vi "THzTimeScan_830_PSD_TA_170120.vi"(0 "input":T1={"Step Number"=0, "Step"=0.0, "Start Position"=0.0, "Time-out"=0, "Lockin Address"="", "Short term \nAverage#"=0, 0, "ESP300 Axis"=0, "Value"="", "Delay"=0.0, "Delay2"=0.0, "savepath"=path "", "Power meter"={"ConexPSD Reference"=refnum, "error out"={"status"=FALSE, "code"=0, "source"=""}, "Component ID"=1}}) -> (1 "loop stop":bool, 2 "x-axis":sgl[](array[numeric]), 3 "y-axis":dbl[](array[numeric]), 4 "ext. out":cluster{dbl[], dbl[], dbl[], dbl[], string[]})   [LabVIEW 2010]
uses:
  <vilib>/Utility/file.llb/Write To Spreadsheet File (string).vi
  C:/Users/NBTP/Desktop/Tai Anh/5. Tools Project/LabVIEW/노트북LabVIEW/THz Time/THz Time(SR830_VC_CONEXAGP_nPt_Shot202_2Pt__LGS/Dll/Newport.CONEXPSD.CommandInterface.DLL
  5. Tools Project/LabVIEW/노트북LabVIEW/THz Time/THz Time(SR830_VC_CONEXAGP_nPt_Shot202_2Pt__LGS/Dll/Newport.CONEXPSD.CommandInterface.DLL
panel:
  out "Y position":dbl(graph)
  out "X position":dbl(graph)
  out "Power":dbl(graph)
  out "Y pos.":dbl
  out "X pos.":dbl
  out "Pow.":dbl
  out "Array":dbl[](array[numeric])
  out "String":string
  out "Read position":bool
  out "Ask position":bool
  out "Move delay":bool
  out "Read830":bool
  out "Command":string
  out "THz Signal Graph":dbl(graph)
  in  "loop stop":bool
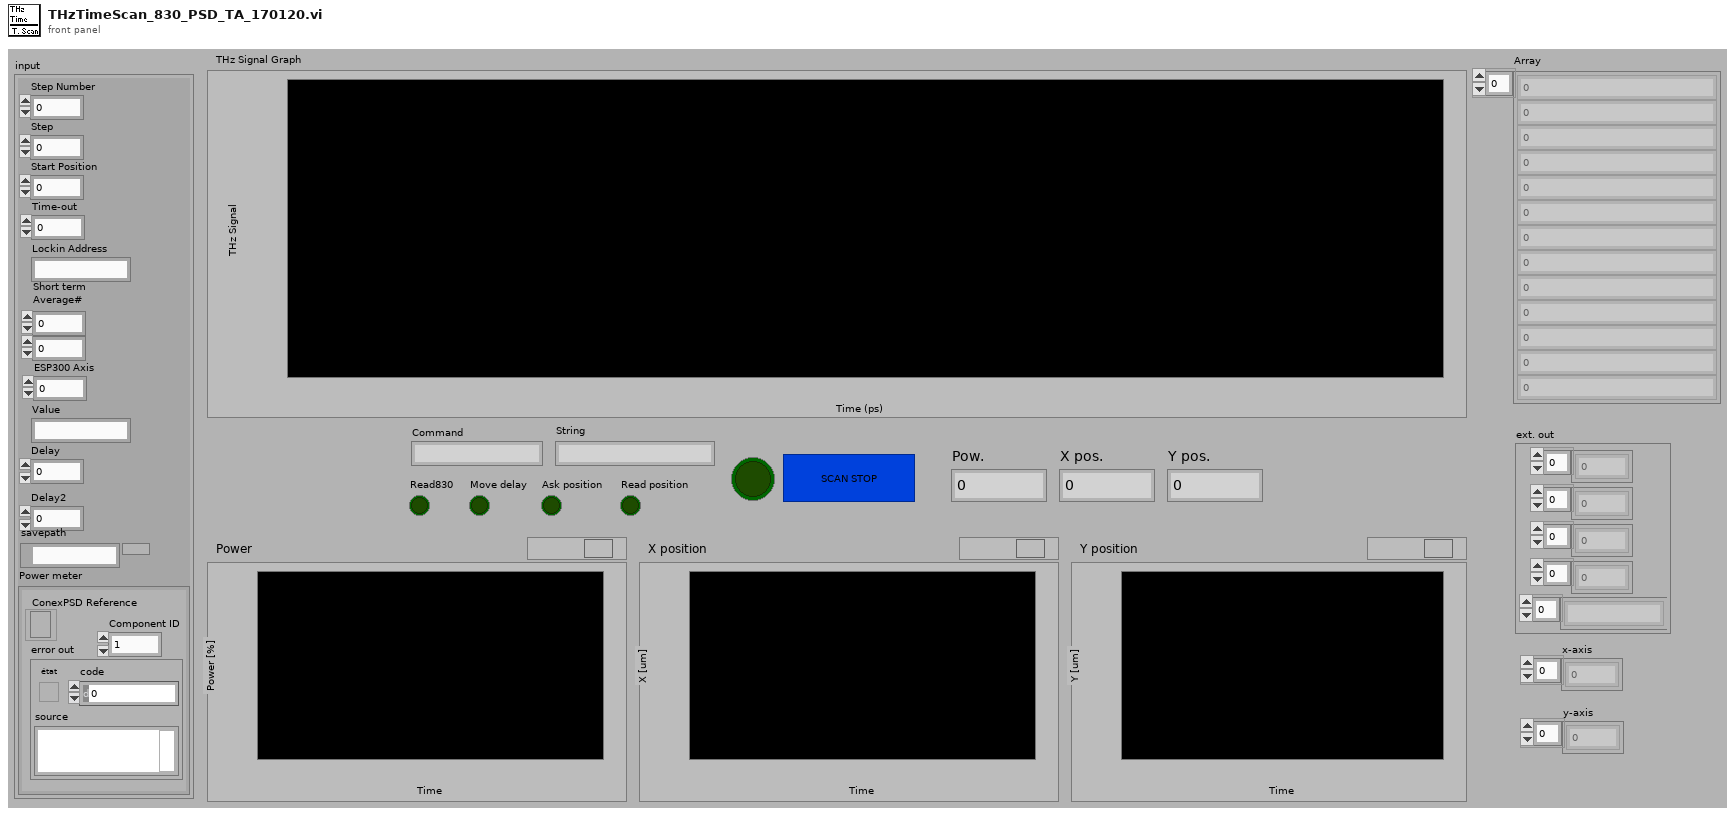
[diagram p1: front panel]
types:
  T1 = cluster{"Step Number":i32, "Step":sgl, "Start Position":sgl, "Time-out":i32, "Lockin Address":string, "Short term \nAverage#":i8, i32, "ESP300 Axis":i8, "Value":string, "Delay":dbl, "Delay2":dbl, "savepath":path, "Power meter":cluster{"ConexPSD Reference":refnum<k24>, "error out":errorcluster, "Component ID":i32}}
  T2 = cluster{"ConexPSD Reference":refnum<k24>, "error out":errorcluster, "Component ID":i32}
  T3 = cluster{"PositionX":dbl, "PositionY":dbl, "LaserPower":dbl}
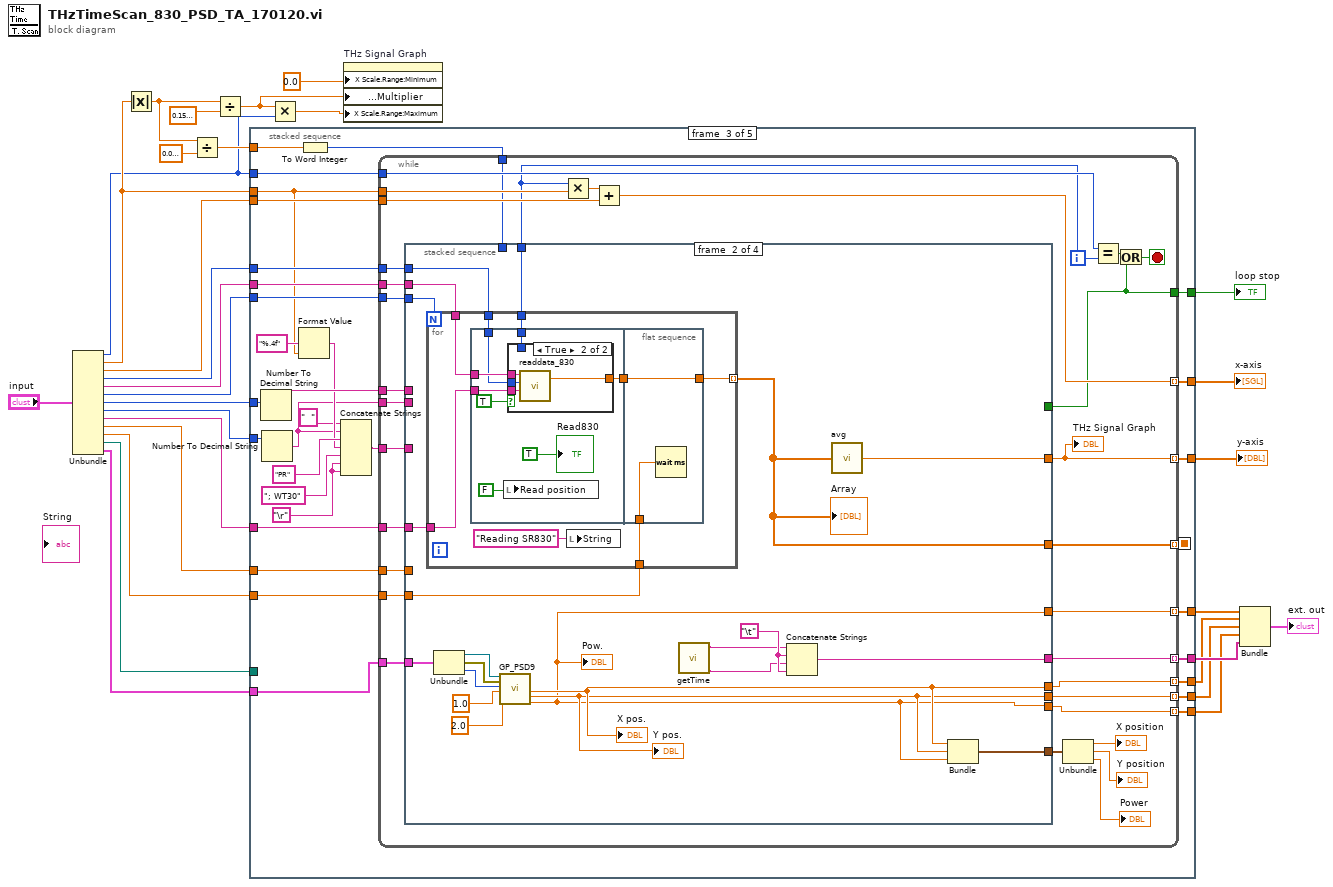
[diagram p0: block diagram]
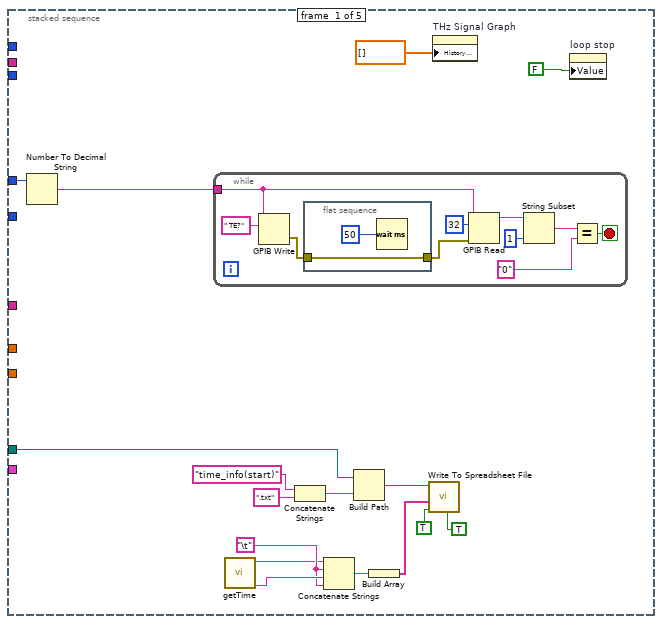
[diagram p2: hidden frame]
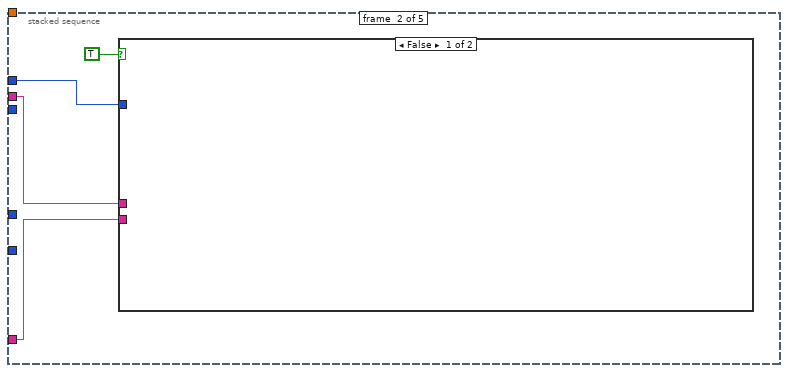
[diagram p3: hidden frame]
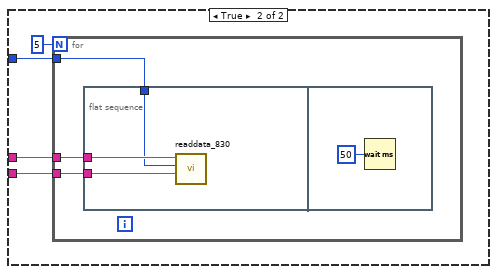
[diagram p4: hidden frame]
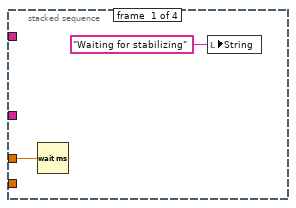
[diagram p5: hidden frame]
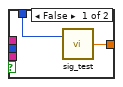
[diagram p6: hidden frame]
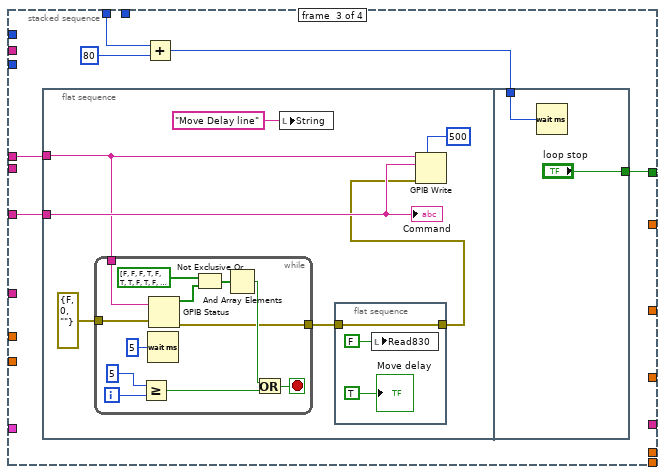
[diagram p7: hidden frame]
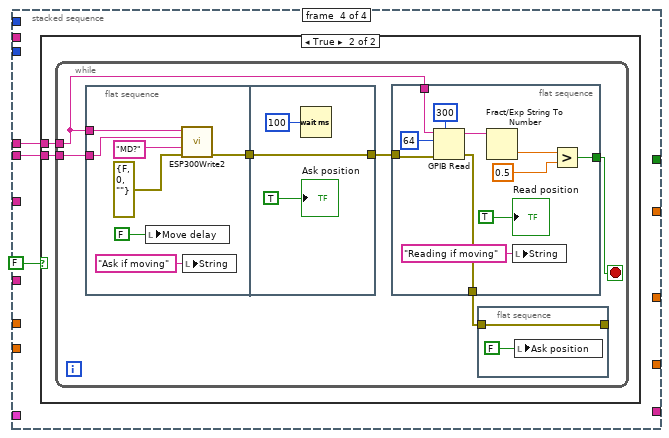
[diagram p8: hidden frame]
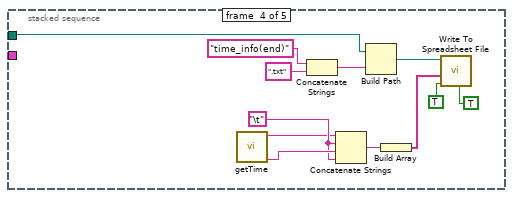
[diagram p10: hidden frame]
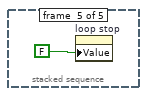
[diagram p11: hidden frame]
diagram:
  n1 = Unbundle("input") -> ("Step Number"=w2:i32, "Step"=w23:sgl, "Start Position"=w22:sgl, "Time-out"=w21:i32, "Lockin Address"=w20:string, "Short term \nAverage#"=w13:i8, w19:i32, "ESP300 Axis"=w18:i8, "Value"=w17:string, "Delay"=w12:dbl, "Delay2"=w11:dbl, "savepath"=w10:path, "Power meter"=w9:T2)
  n2 = Absolute Value(x=w23) -> (abs(x)=w26:sgl)
  n3 = Divide(x=w26, y=sgl 0.004) -> (x/y=w24:sgl)
  n4 = Divide(x=w26, y=sgl 0.15) -> (x/y=w15:sgl)
  n5 = stacked-sequence {
    seq-local: [_ _ w81 _ _] -> [_ _ _ _ _]
    tunnel: w22 -> [_ _ w105 _ _]
    tunnel: w21 -> [_ w62 w104 _ _]
    tunnel: w20 -> [_ w61 w103 _ _]
    tunnel: w13 -> [_ _ w102 _ _]
    tunnel: w19 -> [w44 _ w97 _ _]
    tunnel: w18 -> [_ _ w95 _ _]
    tunnel: w17 -> [_ w60 w87 _ _]
    tunnel: [_ _ w101 _ _] -> w30
    tunnel: [_ _ w100 _ _] -> w29
    tunnel: [_ _ w99 _ _] -> w28
    tunnel: w23 -> [_ _ w93 _ _]
    tunnel: w2 -> [_ _ w98 _ _]
    tunnel: w24 -> [_ _ w92 _ _]
    tunnel: w12 -> [_ _ w83 _ _]
    tunnel: w11 -> [_ _ w82 _ _]
    tunnel: w10 -> [w31 _ _ w249 _]
    tunnel: w9 -> [_ _ w79 _ _]
    tunnel: [_ _ w78 _ _] -> w8
    tunnel: [_ _ w77 _ _] -> w7
    tunnel: [_ _ w76 _ _] -> w6
    tunnel: [_ _ w75 _ _] -> w5
    tunnel: [_ _ w74 _ _] -> w4
    frame #0 {
      w34 = "\t"
      n6 = Number To Decimal String(number=w44) -> (decimal integer string=w43:string)  [unwired: 1 in]
      n7 = while {
        tunnel: w43 -> [w49]
        stop <- w54 stop-if-true
        n8 = GPIB Write(0:w49, 1:" TE?" ("data")) -> (6:w48:errorcluster)  [unwired: 3 in, 1 out]
        n9 = flat-sequence {
          tunnel: w48 -> [w58]
          tunnel: [w58] -> w47
          frame #0 {
            n10 = Wait (ms)(milliseconds to wait=u32 50) -> ()  [unwired: 1 out]
          }
        }
        n11 = GPIB Read(0:w49, 1:32 ("byte count"), 3:w47) -> (5:w53:string)  [unwired: 2 in, 2 out]
        n12 = String Subset(string=w53, length (rest)=1 ("offset (0)")) -> (substring=w51:string)  [unwired: 1 in]
        n13 = Equal?(x=w51, y="0") -> (x = y?=w54:bool)
      }
      n14 = call "getTime.vi"() -> ("시간"=w35:string, "날짜"=w33:string)  [unwired: 10 in]
      n15 = Concatenate Strings("time_info(start)" ("string"), ".txt" ("string")) -> (w41:string)
      n16 = Concatenate Strings(w33, w34, w35, w34) -> (w32:string)
      n17 = Build Path(base path=w31, name or relative path=w41) -> (appended path=w38:path)
      n18 = Build Array(w32) -> (w37:string[])
      n19 = call-poly <vilib>:"Write To Spreadsheet File.vi"("transpose? (no:F)"=TRUE ("transpose?\n(no:F)"), "append to file? (new file:F)"=TRUE ("transpose?\n(no:F)"), "1D data"=w37, "file path (dialog if empty)"=w38) -> ()  [unwired: 4 in, 1 out]
      n20 = property on="THz Signal Graph" class="WFChart (strict)"("History Data"=dbl[] []) -> ()  [unwired: 2 in, 2 out]
      n21 = property on="loop stop" class="Bool (strict)"("Value"=FALSE) -> ()  [unwired: 2 in, 2 out]
    }
    frame #1 {
      n22 = case shown="False" TRUE {
        tunnel: w62 -> [_ w65]
        tunnel: w61 -> [_ w64]
        tunnel: w60 -> [_ w63]
        frame False {
        }
        frame True {
          n23 = for {
            N: 5 -> [_]
            tunnel: w64 -> [w69]
            tunnel: w63 -> [w68]
            tunnel: w65 -> [w67]
            n24 = flat-sequence {
              tunnel: w69 -> [w72]
              tunnel: w68 -> [w71]
              tunnel: w67 -> [w70]
              frame #0 {
                n25 = call "readdata_830.vi"("Command"=w71, "timeout"=w70, "Lockin Address"=w72) -> ()  [unwired: 1 in, 2 out]
              }
              frame #1 {
                n26 = Wait (ms)(milliseconds to wait=u32 50) -> ()  [unwired: 1 out]
              }
            }
          }
        }
      }
    }
    frame #2 {
      w86 = "\r"
      n27 = Number To Decimal String(number=w97) -> (decimal integer string=w96:string)  [unwired: 1 in]
      n28 = Number To Decimal String(number=w95) -> (decimal integer string=w84:string)  [unwired: 1 in]
      n29 = Format Value(format string="%.4f", value (0)=w93) -> (output string=w89:string)  [unwired: 1 in]
      n30 = To Word Integer(number=w92) -> (16bit integer=w91:i16)
      n31 = Concatenate Strings("  " ("string"), w84, "PR" ("Substring"), w89, "; WT30" ("string"), w86, w86) -> (w80:string)
      n32 = while {
        tunnel: [w121] -> w101
        tunnel: [w127] -> w99 mode=indexing
        tunnel: [w133] -> w100 mode=indexing
        tunnel: w98 -> [w132]
        tunnel: w93 -> [w131]
        tunnel: w105 -> [w130]
        tunnel: w104 -> [w122]
        tunnel: w103 -> [w129]
        tunnel: w102 -> [w128]
        tunnel: w96 -> [w126]
        tunnel: w80 -> [w125]
        tunnel: w91 -> [w124]
        tunnel: w87 -> [w123]
        tunnel: w84 -> [w120]
        tunnel: w83 -> [w119]
        tunnel: w82 -> [w118]
        tunnel: [w117] -> w81 mode=indexing
        tunnel: w79 -> [w115]
        tunnel: [w114] -> w75 mode=indexing
        tunnel: [w113] -> w76 mode=indexing
        tunnel: [w112] -> w74 mode=indexing
        tunnel: [w111] -> w78 mode=indexing
        tunnel: [w110] -> w77 mode=indexing
        i -> [w116]
        stop <- w136 stop-if-true
        n33 = stacked-sequence {
          tunnel: w129 -> [_ w157 _ _]
          tunnel: [_ w159 _ _] -> w127
          tunnel: w128 -> [_ w160 _ _]
          tunnel: w126 -> [_ _ w189 w217]
          tunnel: w125 -> [_ _ w190 _]
          tunnel: w124 -> [_ _ w188 _]
          tunnel: w123 -> [_ w158 _ _]
          tunnel: w122 -> [_ w156 _ _]
          tunnel: [_ _ w185 _] -> w121
          tunnel: w120 -> [_ _ _ w216]
          tunnel: w119 -> [w138 _ _ _]
          tunnel: w118 -> [_ w155 _ _]
          tunnel: [_ w154 _ _] -> w117
          tunnel: w116 -> [_ w153 _ _]
          tunnel: w115 -> [_ w146 _ _]
          tunnel: [_ w139 _ _] -> w111
          tunnel: [_ w145 _ _] -> w110
          tunnel: [_ w141 _ _] -> w113
          tunnel: [_ w140 _ _] -> w114
          tunnel: [_ w139 _ _] -> w112
          tunnel: [_ w144 _ _] -> w109
          frame #0 {
            n34 = Wait (ms)(milliseconds to wait=w138) -> ()  [unwired: 1 out]
            n35 = local write "String"("Waiting for stabilizing" ("String")) -> ()
          }
          frame #1 {
            w147 = "\t"
            n36 = for {
              N: w160 -> [_]
              tunnel: w157 -> [w165]
              tunnel: w156 -> [w168]
              tunnel: [w167] -> w154 mode=indexing
              tunnel: w158 -> [w166]
              tunnel: w155 -> [w162]
              tunnel: w153 -> [w161]
              n37 = flat-sequence {
                tunnel: w168 -> [w172]
                tunnel: w166 -> [w173]
                tunnel: w165 -> [w174]
                tunnel: [w171] -> w163
                tunnel: w161 -> [w169]
                tunnel: [w184] -> w167
                tunnel: w163 -> [w184]
                tunnel: w162 -> [w183]
                frame #0 {
                  n38 = local write "Read position"(FALSE ("Read position")) -> ()
                  n39 = case shown="True" TRUE {
                    tunnel: w174 -> [_ w182]
                    tunnel: w173 -> [_ w181]
                    tunnel: w172 -> [_ w180]
                    tunnel: [w178 w179] -> w171
                    tunnel: w169 -> [w177 _]
                    frame False {
                      n40 = call "sig_test.vi"("index (row)"=w177) -> ("element"=w178:dbl)  [unwired: 1 in]
                    }
                    frame True {
                      n41 = call "readdata_830.vi"("Command"=w181, "timeout"=w180, "Lockin Address"=w182) -> ("Data"=w179:dbl)  [unwired: 1 in, 1 out]
                    }
                  }
                  "Read830" <- TRUE ("Read830")
                }
                frame #1 {
                  n42 = Wait (ms)(milliseconds to wait=w183) -> ()  [unwired: 1 out]
                }
              }
              n43 = local write "String"("Reading SR830" ("String")) -> ()
            }
            "Array" <- w154
            n44 = Unbundle(w146) -> ("ConexPSD Reference"=w152:refnum<k24>, "error out"=w151:errorcluster, "Component ID"=w150:i32)
            n45 = call "GP_PSD9.vi"("ConexPSD Reference"=w152, "error out"=w151, "Component ID"=w150, "Adress"=1.0, "shot average"=2.0) -> ("PositionX"=w141:dbl, "PositionY"=w140:dbl, "LaserPower"=w139:dbl)  [unwired: 8 in, 4 out]
            "Pow." <- w139
            "X pos." <- w141
            "Y pos." <- w140
            n46 = call "getTime.vi"() -> ("시간"=w142:string, "날짜"=w143:string)  [unwired: 10 in]
            n47 = Concatenate Strings(w143, w147, w142, w147) -> (w145:string)
            n48 = call "avg.vi"("Array"=w154) -> ("Numeric"=w159:dbl)
            n49 = Bundle("PositionX"=w141, "PositionY"=w140, "LaserPower"=w139) -> (w144:T3)  [unwired: 1 in]
          }
          frame #2 {
            n50 = flat-sequence {
              tunnel: w190 -> [w197]
              tunnel: w189 -> [w195]
              tunnel: w187 -> [w213]
              tunnel: ["loop stop"] -> w185
              frame #0 {
                n51 = while {
                  tunnel: errorcluster {"status"=FALSE, "code"=0, "source"=""} ("error in (no error)") -> [w212]
                  tunnel: [w202] -> w192
                  tunnel: w195 -> [w201]
                  i -> [w211]
                  stop <- w208 stop-if-true
                  n52 = Greater Or Equal?(x=5, y=w211) -> (x >= y?=w209:bool)
                  n53 = Wait (ms)(milliseconds to wait=u32 5) -> ()  [unwired: 1 out]
                  n54 = GPIB Status(0:w201, 1:w212) -> (2:w206:bool[], 5:w202:errorcluster)  [unwired: 2 out]
                  n55 = Not Exclusive Or(1:w206, 2:bool[] [FALSE, FALSE, FALSE, TRUE, FALSE, TRUE, TRUE, FALSE, TRUE, FALSE, FALSE, FALSE, FALSE, FALSE, FALSE, FALSE] ("status 2")) -> (0:w205:bool[])
                  n56 = And Array Elements(Boolean array=w205) -> (logical AND=w204:bool)
                  n57 = Or(x=w204, y=w209) -> (x .or. y?=w208:bool)
                }
                n58 = local write "String"("Move Delay line" ("String")) -> ()
                n59 = flat-sequence {
                  tunnel: [w200] -> w193
                  tunnel: w192 -> [w200]
                  frame #0 {
                    n60 = local write "Read830"(FALSE ("Read830")) -> ()
                    "Move delay" <- TRUE ("Move delay")
                  }
                }
                n61 = GPIB Write(0:w195, 1:w197, 3:w193, 4:500 ("timeout ms (488.2 global)")) -> ()  [unwired: 1 in, 2 out]
                "Command" <- w197
              }
              frame #1 {
                n62 = Wait (ms)(milliseconds to wait=w213) -> ()  [unwired: 1 out]
              }
            }
            n63 = Add(x=w188, y=i16 80) -> (x+y=w187:i16)
          }
          frame #3 {
            n64 = case shown="True" FALSE {
              tunnel: w217 -> [_ w219]
              tunnel: w216 -> [_ w218]
              frame False {
              }
              frame True {
                n65 = while {
                  tunnel: w219 -> [w221]
                  tunnel: w218 -> [w225]
                  stop <- w223 stop-if-true
                  n66 = flat-sequence {
                    tunnel: w225 -> [w239]
                    tunnel: w221 -> [w242]
                    tunnel: [w243] -> w222
                    tunnel: [w248] -> w224
                    tunnel: w222 -> [w248]
                    frame #0 {
                      n67 = local write "Move delay"(FALSE ("Move delay")) -> ()
                      n68 = call "ESP300Write2.vi"("error in (no error)"=errorcluster {"status"=FALSE, "code"=0, "source"=""}, "Command"="MD?", "ESP300 Channel"=w239, "ESP300 Address"=w242) -> ("error out"=w243:errorcluster)  [unwired: 3 in]
                      n69 = local write "String"("Ask if moving" ("String")) -> ()
                    }
                    frame #1 {
                      n70 = Wait (ms)(milliseconds to wait=u32 100) -> ()  [unwired: 1 out]
                      "Ask position" <- TRUE ("Ask position")
                    }
                  }
                  n71 = flat-sequence {
                    tunnel: w224 -> [w238]
                    tunnel: [w235] -> w223
                    tunnel: w221 -> [w231]
                    tunnel: [w229] -> w220
                    frame #0 {
                      n72 = GPIB Read(0:w231, 1:64 ("byte count"), 3:w238, 4:300 ("timeout ms (488.2 global)")) -> (5:w234:string, 7:w229:errorcluster)  [unwired: 1 in, 1 out]
                      n73 = Fract/Exp String To Number(string=w234) -> (number=w233:dbl)  [unwired: 3 in, 1 out]
                      n74 = local write "String"("Reading if moving" ("String")) -> ()
                      n75 = Greater?(x=w233, y=0.5) -> (0:w235:bool)
                      "Read position" <- TRUE ("Read position")
                    }
                  }
                  n76 = flat-sequence {
                    tunnel: [w227] -> _
                    tunnel: w220 -> [w227]
                    frame #0 {
                      n77 = local write "Ask position"(FALSE ("Ask position")) -> ()
                    }
                  }
                }
              }
            }
          }
        }
        "THz Signal Graph" <- w127
        n78 = Multiply(x=w116, y=w131) -> (x*y=w134:sgl)
        n79 = Add(x=w134, y=w130) -> (x+y=w133:sgl)
        n80 = Unbundle(w109) -> ("PositionX"=→"X position":dbl, "PositionY"=→"Y position":dbl, "LaserPower"=→"Power":dbl)
        n81 = Equal?(x=w132, y=w116) -> (x = y?=w135:bool)
        n82 = Or(x=w135, y=w121) -> (x .or. y?=w136:bool)
      }
    }
    frame #3 {
      w252 = "\t"
      n83 = call "getTime.vi"() -> ("시간"=w253:string, "날짜"=w251:string)  [unwired: 10 in]
      n84 = Concatenate Strings("time_info(end)" ("string"), ".txt" ("string")) -> (w259:string)
      n85 = Concatenate Strings(w251, w252, w253, w252) -> (w250:string)
      n86 = Build Path(base path=w249, name or relative path=w259) -> (appended path=w256:path)
      n87 = Build Array(w250) -> (w255:string[])
      n88 = call-poly <vilib>:"Write To Spreadsheet File.vi"("transpose? (no:F)"=TRUE ("transpose?\n(no:F)"), "append to file? (new file:F)"=TRUE ("transpose?\n(no:F)"), "1D data"=w255, "file path (dialog if empty)"=w256) -> ()  [unwired: 4 in, 1 out]
    }
    frame #4 {
      n89 = property on="loop stop" class="Bool (strict)"("Value"=FALSE) -> ()  [unwired: 2 in, 2 out]
    }
  }
  "loop stop" <- w30
  "x-axis" <- w29
  "y-axis" <- w28
  n90 = Multiply(x=w15, y=w2) -> (x*y=w14:sgl)
  n91 = property on="THz Signal Graph" class="WFChart (strict)"("X Scale.Range:Minimum"=0.0, "X Scale.Offset and Multiplier:Multiplier"=w15, "X Scale.Range:Maximum"=w14) -> ()  [unwired: 2 in, 2 out]
  n92 = Bundle(w8, w6, w5, w4, w7) -> (→"ext. out":cluster{dbl[], dbl[], dbl[], dbl[], string[]})  [unwired: 1 in]
